vi "2d-color-to-1d-color.vi"(10 "Real Matrix in":T1, 11 "image data":T2) -> (3 "Real Matrix out 2":dbl[](array[numeric]))   [LabVIEW 2016]
uses:
  <vilib>/picture/picture.llb/imagedata.ctl
  <vilib>/Analysis/Matrix/Datatypes/RealMatrix.ctl
  <vilib>/Analysis/Matrix/NI_Matrix.lvlib
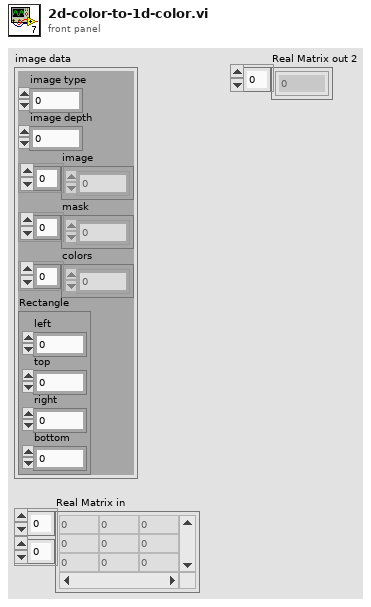
[diagram p1: front panel]
types:
  T1 = typedef "NI_Matrix.lvlib/RealMatrix.ctl" = dbl[][]
  T2 = typedef "imagedata.ctl" = cluster{"image type":i32, "image depth":i32, "image":u8[], "mask":u8[], "colors":u32[], "Rectangle":cluster{"left":i16, "top":i16, "right":i16, "bottom":i16}}
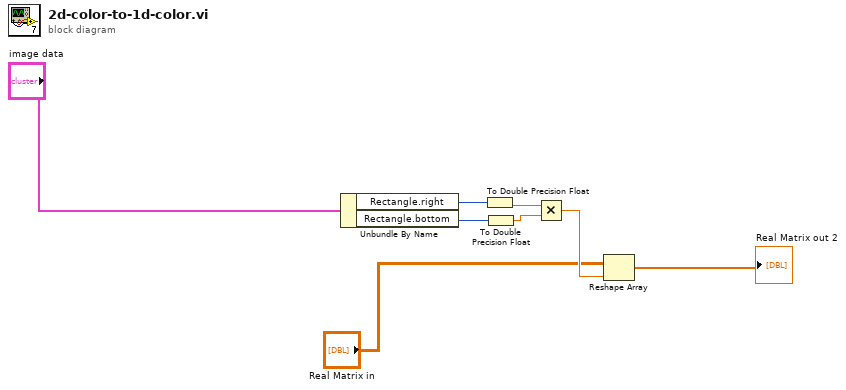
[diagram p0: block diagram]
diagram:
  n1 = Unbundle By Name("image data") -> ("Rectangle.right"=w6:i16, "Rectangle.bottom"=w7:i16)
  n2 = To Double Precision Float(number=w6) -> (double precision float=w5:dbl)
  n3 = To Double Precision Float(number=w7) -> (double precision float=w4:dbl)
  n4 = Multiply(x=w5, y=w4) -> (x*y=w8:dbl)
  n5 = Reshape Array("Real Matrix in", w8) -> (→"Real Matrix out 2":dbl[])
